vi "Write configuration.vi"(8 "error in (no error)":errorcluster, 11 "StageSPIM in":refnum<class "StageSPIM.lvclass">) -> (0 "error out":errorcluster, 3 "StageSPIM out":refnum<class "StageSPIM.lvclass">)   [LabVIEW 2012, in "StageSPIM.lvclass"]
doc: "Writes the configuration cluster into the configuration file. Configuration file is XML-based. It's name is <component ID>.xml"
uses:
  StageSPIM.lvclass
  <vilib>/Distrio/Murmex/Murmex/Murmex.lvclass
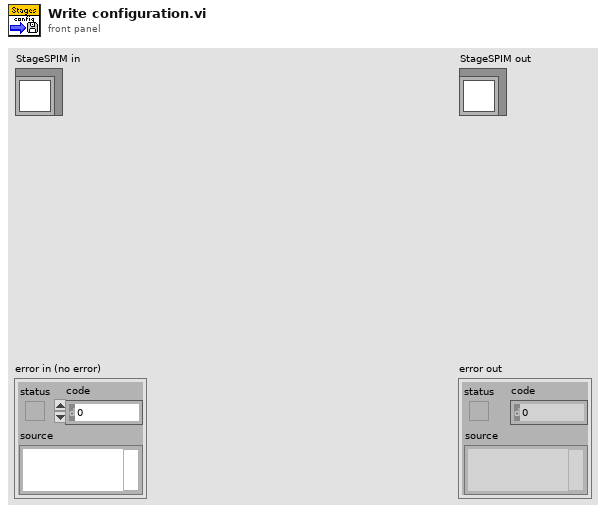
[diagram p1: front panel]
types:
  T1 = typedef "StageSPIM.lvclass/configuration_cluster.ctl" = cluster{"Port":T2, "Baudrate":T3, "Update frequency":dbl[unit], "S/N Master controller":string, "Interface":T4, "soft min limit":dbl[], "soft max limit":dbl[], "startup speedA":dbl[unit], "startup speedX":dbl[unit], "startup speedY":dbl[unit], "startup speedZ":dbl[unit], "startup speedFocus":dbl[unit], "autofocus ID":string}
  T2 = typedef "StageSPIM.lvclass/port_control.ctl" = i32
  T3 = typedef "StageSPIM.lvclass/baud_rate_control.ctl" = u16
  T4 = typedef "StageSPIM.lvclass/connection_type.ctl" = enum16{"RS232", "RS232 DaisyChain", "USB", "USB_DaisyChain"}
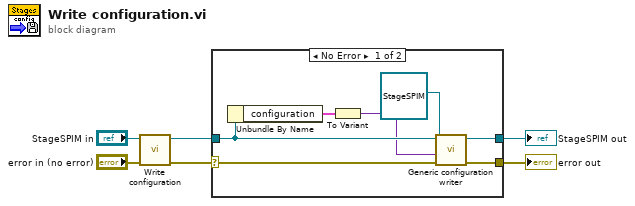
[diagram p0: block diagram]
diagram:
  n1 = call-parent "Write configuration.vi"("error in (no error)"="error in (no error)", "Murmex in"="StageSPIM in") -> ("error out"=w4:errorcluster, "Murmex out"=w3:refnum<class "StageSPIM.lvclass">)  [unwired: 8 in]
  n2 = case shown="No Error" w4 {
    selector: w4 -> [w10 w14]
    tunnel: w3 -> [w9 w15]
    tunnel: [w12 w15] -> w2
    tunnel: [w11 w14] -> w1
    frame No Error {
      n3 = Unbundle By Name(w9) -> ("configuration"=w8:T1)
      n4 = To Variant(anything=w8) -> (Variant=w7:variant)
      n5 = call <vilib>:"Generic configuration writer.vi"("error in (no error)"=w10, 9:w7, 10:refnum<class "StageSPIM.lvclass"> refnum ("StageSPIM.lvclass"), "Murmex in"=w9) -> ("error out"=w11:errorcluster, "Murmex out"=w12:refnum<class "StageSPIM.lvclass">)  [unwired: 6 in]
    }
    frame Error {
    }
  }
  "error out" <- w1
  "StageSPIM out" <- w2
